vi "Total Analysis.vi"(6 "ROIIndex":i32, 7 "Algorithm":T1, 8 "error in":errorcluster, 9 "ROIList":string[][](array[string]), 10 "AlgParameter":string, 11 "Img in":T2) -> (0 "error out":errorcluster, 1 "DetectResult":variant, 2 "ResultOut":string[][](array[string]), 3 "Img out":T2)   [LabVIEW 2019]
uses:
  <vilib>/vision/Image Controls.llb/IMAQ Image.ctl
  Controls/V_Analysis_Type.ctl
  Controls/Analysis_Setting.ctl
  Ctrl/ROIDataType.ctl
  Controls/Parameter.ctl
  Controls/Color Pattern Match/Analysis Color Pattern Match Parameter.ctl
  Controls/Color Pattern Match/Analysis Color Pattern Match Result.ctl
  Controls/Parttern Match/Analysis_PatternMatch_Parameter.ctl
  Controls/ShapeDectect/Analysis_ShapeDectect_Parameter.ctl
  a7e08b04-c8a4-4d17-8d88-fa481432bc0a.vi
  bf7b5f5d-5c07-4b16-8f99-98f9c9cab738.vi
  dd62c550-2db8-45b5-a3de-447688dd18ca.vi
  c9a32d4f-7d2d-4bd1-920f-33aa71ed714f.vi
  4b400e5f-8bf9-44aa-89bd-445ffc1e469d.vi
  <vilib>/JDP Science/JSONtext/JSON text to Variant.vi
  <vilib>/vision/NI_Vision_Development_Module.lvlib
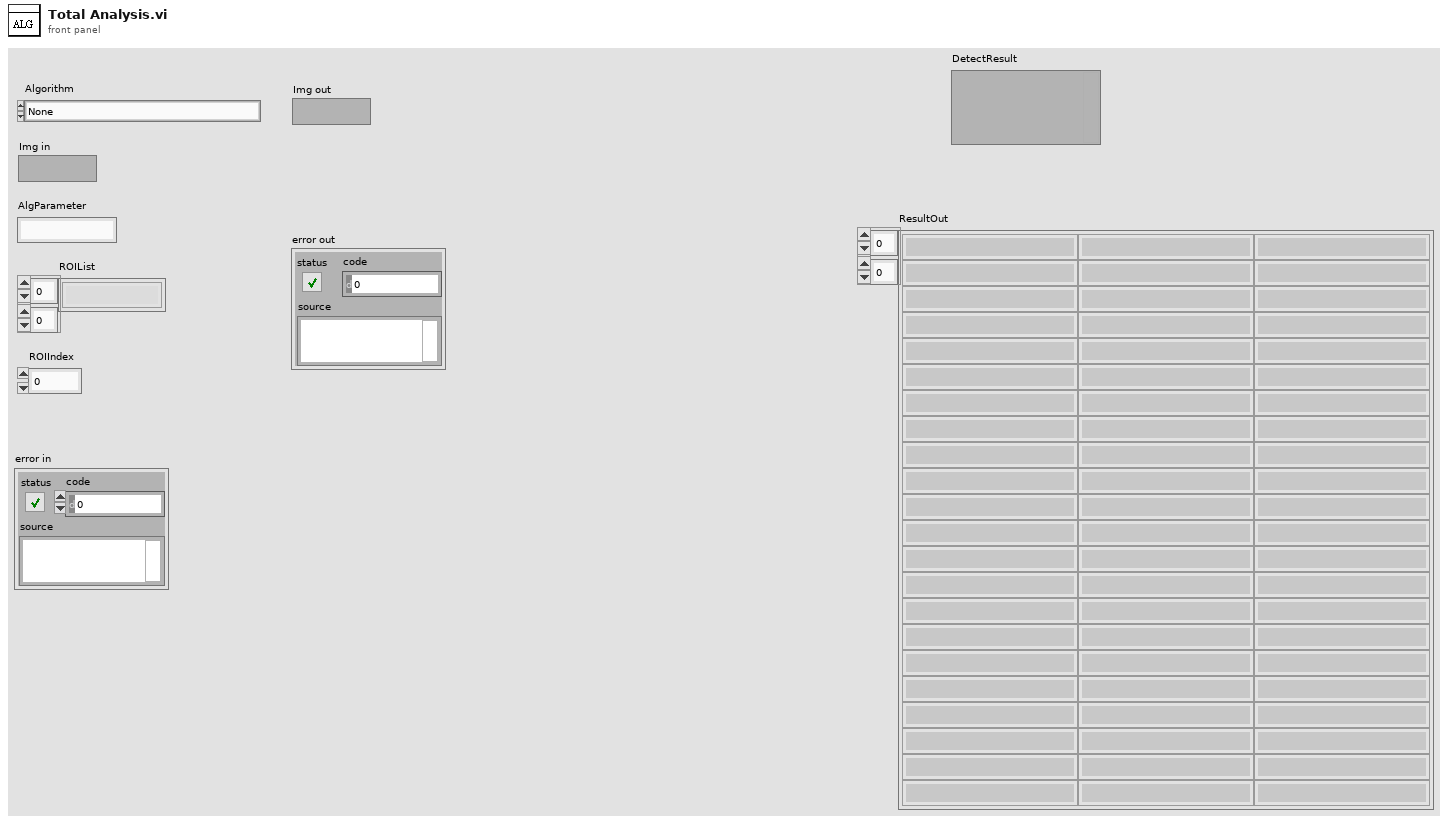
[diagram p1: front panel]
types:
  T1 = typedef "V_Analysis_Type.ctl" = enum16{"None", "C_Color Pattern Matching", "G_PatternMatching", "G_ShapeDectect", "G_GeometricMatch"}
  T2 = typedef "IMAQ Image.ctl" = refnum<image>
  T3 = typedef "Parameter.ctl" = enum16{"Initialize", "Write", "Read", "WriteAll", "Save", "Load"}
  T4 = typedef "ROIDataType.ctl" = cluster{"Global Rectangle":i32[], "Contours":cluster{"Contour Type":u32, "ROI Type":u32, "Points":i32[]}[]}
  T5 = typedef "Analysis Color Pattern Match Parameter.ctl" = cluster{"IgnoreBlack And White":enum16{"Disable", "IgnoreBlack", "IgnoreWhite", "IgnoreBlack And White"}, "Match Saturation Threshold":i32, "Minimum Match Score":i32, "Color Score Weight":i32, "Color Sensitivity":u32, "Search Strategy":u32, "Match Offset":cluster{"X":dbl, "Y":dbl}, "Number of Matches to Find":i32, "AngleRange+/-":dbl, "Sub-Pixel Accuracy":bool, "ROI Descriptor":T6, "TemplatePath":string, "Match Mode":enum16{"Shift Invariant", "Rotation Invariant"}}
  T6 = typedef "ROI Descriptor" = cluster{"Global Rectangle":i32[], "Contours":cluster{"ID":enum32{"External", "Internal"}, "Type":u32, "Coordinates":i32[]}[]}
  T7 = typedef "Analysis_ShapeDectect_Parameter.ctl" = cluster{"Enum_ShapeType":enum16{"Circles", "Ellipses", "Lines", "Rectangles"}, "MaxParticle":i32, "Descriptor":cluster{"Set 1":dbl, "Set 2":dbl, "Set 3":dbl, "Set 4":dbl}, "Match Options":cluster{"Rotation":bool, "Scale":bool, "Occlusion":bool, "Range Settings":cluster{"Match Constraints":u32, "Min":dbl, "Max":dbl}[]}, "Curve Parameters":cluster{"Extraction Mode":u32, "Edge Threshold":i32, "Edge Filter Size":u32, "Min Length":i32, "Row Search Step Size":i32, "Col Search Step Size":i32, "Max Endpoint Gap":i32, "Closed":bool, "Subpixel":bool}, " score":dbl}
  T8 = typedef "Analysis_Setting.ctl" = cluster{"PreProcess":T1, "Parameter":string}
  T9 = typedef "ParameterData.ctl" = cluster{"Rotate Angle":dbl, "Rotate?":bool, "Calibration File Path":string, "Cal?":bool}
  T10 = typedef "Image Type" = u32
  T11 = typedef "Analysis Color Pattern Match Result.ctl" = cluster{"Number of Matches":i32, "Matches out":cluster{"Position":cluster{"x":sgl, "y":sgl}, "Angle":sgl, "Scale":sgl, "Score":sgl, "Bounding Box":cluster{"x":sgl, "y":sgl}[]}[], "Calibrated Matches":cluster{"Position":cluster{"x":sgl, "y":sgl}, "Angle":sgl, "Scale":sgl, "Score":sgl, "Bounding Box":cluster{"x":sgl, "y":sgl}[]}[], "ROI Descriptor":T6}
  T12 = cluster{"Position":cluster{"x":sgl, "y":sgl}, "Angle":sgl, "Scale":sgl, "Score":sgl, "Bounding Box":cluster{"x":sgl, "y":sgl}[]}[]
  T13 = typedef "Analysis_PatternMatch_Parameter.ctl" = cluster{"Algorithm":i32, "Match Parameters":cluster{"Number of Matches Requested":i32, "Minimum Match Score":sgl, "Angle Ranges":cluster{"Start Angle":sgl, "End Angle":sgl}[]}, "ROI Descriptor":T6, "Advanced Options":cluster{"Item":u16, "Value":dbl}[], "Template path":string, "XOffset":i32, "YOffset":i32}
  T14 = typedef "Analysis_PatternMatch_Result.ctl" = cluster{"Position":cluster{"x":sgl, "y":sgl}, "Angle":sgl, "Scale":sgl, "Score":sgl, "Bounding Box":cluster{"x":sgl, "y":sgl}[]}
  T15 = cluster{"ResultOut":variant, "DectectItem":i32, "Data out":T4}
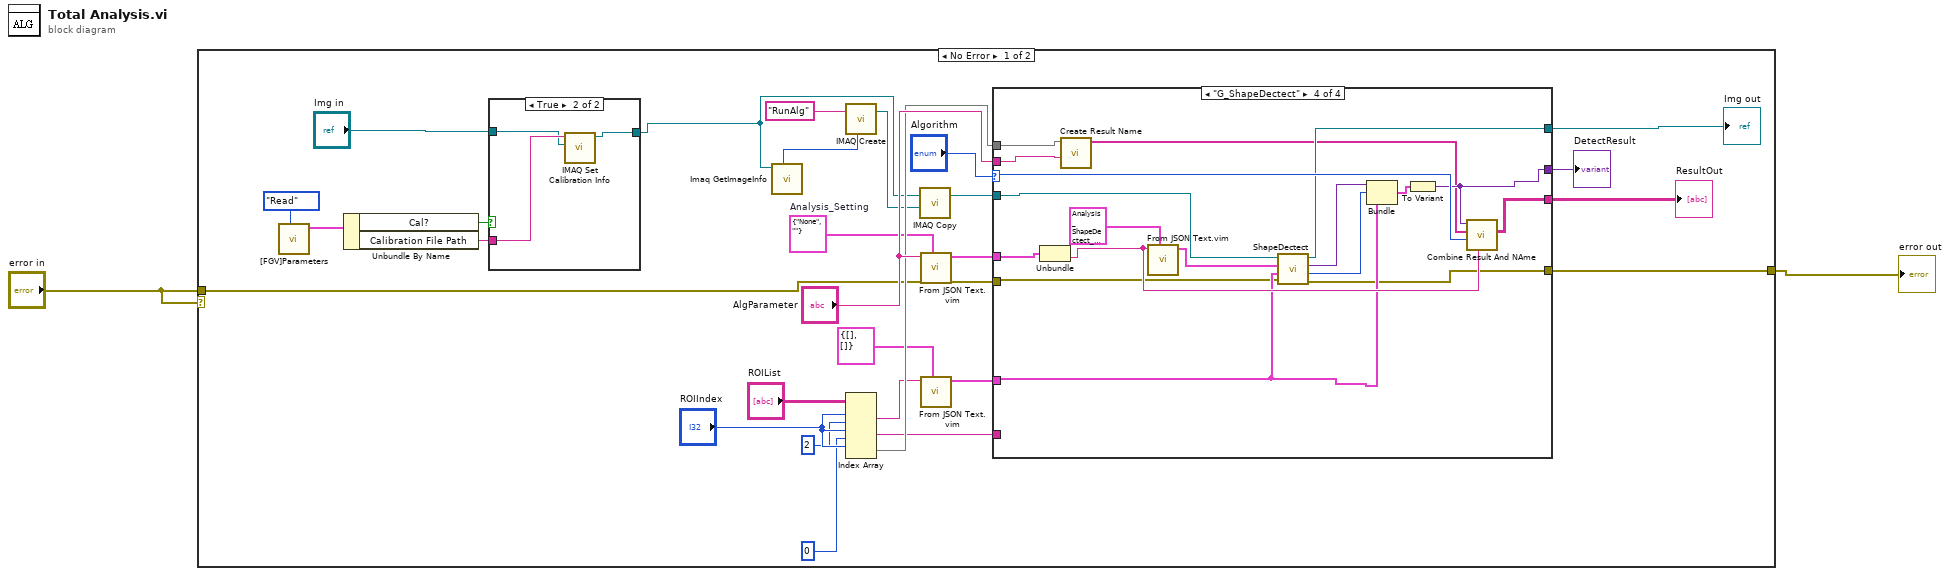
[diagram p0: block diagram]
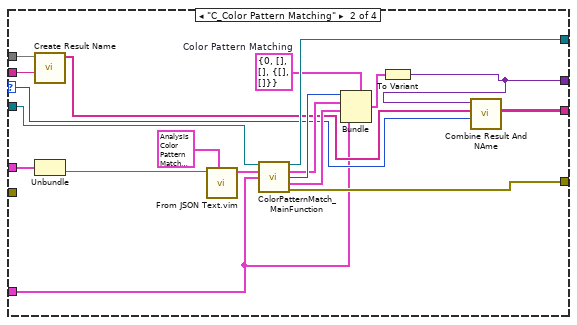
[diagram p4: hidden frame]
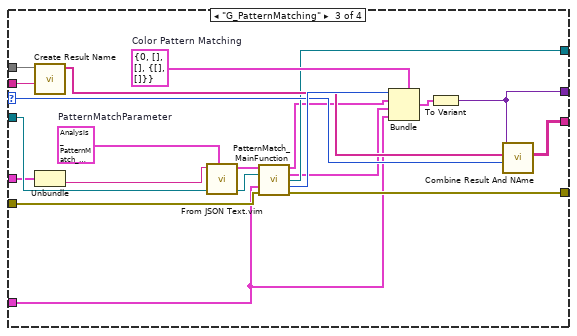
[diagram p5: hidden frame]
diagram:
  n1 = case shown="No Error" "error in" {
    tunnel: [w28 w92] -> w2
    tunnel: "error in" -> [w13 w92]
    frame No Error {
      w14 = T8 {"PreProcess"=enum."None", "Parameter"=""}  # Analysis_Setting
      n2 = call "[FGV]Parameters.vi"("Parameter"=Parameter."Read") -> ("ParameterData Out"=w7:T9)  [unwired: 9 in, 1 out]
      n3 = Unbundle By Name(w7) -> ("Cal?"=w6:bool, "Calibration File Path"=w5:string)
      n4 = case shown="True" w6 {
        tunnel: "Img in" -> [w31 w33]
        tunnel: w5 -> [_ w34]
        tunnel: [w31 w32] -> w3
        frame False {
        }
        frame True {
          n5 = call "IMAQ Set Calibration Info"("Image Dst"=w33, "Image Src"=w34) -> ("Calibrated Image"=w32:T2)  [unwired: 8 in, 1 out]
        }
      }
      n6 = call "Imaq GetImageInfo"("Image"=w3) -> ("Image Type"=w15:T10)  [unwired: 3 in, 7 out]
      n7 = call "IMAQ Create"("Image Name"="RunAlg", "Image Type"=w15) -> ("New Image"=w16:T2)  [unwired: 3 in, 1 out]
      n8 = Index Array(array="ROIList", index (row) #1="ROIIndex", index (col) #1=2 ("disabled index (col)"), index (row) #2="ROIIndex", index (col) #2=0 ("disabled index (col)"), index (row) #3="ROIIndex") -> (element #1=w21:string, element #2=w24:string, element #3=w27:string[])  [unwired: 1 in]
      n9 = call "IMAQ Copy"("Image Dst"=w16, "Image Src"=w3) -> ("Image Dst Out"=w18:T2)  [unwired: 4 in, 1 out]
      n10 = call "From JSON Text.vim"("Data Type and Default Value"=w14, "JSON"="AlgParameter") -> ("Data out"=w25:T8)  [unwired: 8 in, 1 out]
      n11 = call "From JSON Text.vim"("Data Type and Default Value"=T4 {"Global Rectangle"=[], "Contours"=[]} ("ROI DataType"), "JSON"=w21) -> ("Data out"=w22:T4)  [unwired: 8 in, 1 out]
      n12 = case shown="\"G_ShapeDectect\"" "Algorithm" {
        selector: "Algorithm" -> [_ w40 w65 w81]
        tunnel: w18 -> [_ w53 w73 w82]
        tunnel: w22 -> [_ w35 w56 w85]
        tunnel: [_ w52 w61 w80] -> w10
        tunnel: w24 -> [_ _ _ _]
        tunnel: w25 -> [_ w49 w71 w83]
        tunnel: w27 -> [_ w47 w70 w76]
        tunnel: [_ w42 w67 w77] -> w28
        tunnel: "AlgParameter" -> [_ w39 w64 w75]
        tunnel: [_ w38 w60 w78] -> w30
        tunnel: w13 -> [_ _ w59 w84]
        tunnel: [_ w36 w57 w79] -> w11
        frame "None", Default {
        }
        frame "C_Color Pattern Matching" {
          w46 = T11 {"Number of Matches"=0, "Matches out"=[], "Calibrated Matches"=[], "ROI Descriptor"={"Global Rectangle"=[], "Contours"=[]}}  # Color Pattern Matching
          n13 = call "Create Result Name.vi"("AlgSet"=w39, "ROIList"=w47) -> ("AlgResultName"=w41:string[])  [unwired: 9 in]
          n14 = Unbundle(w49) -> ("Parameter"=w51:string)  [unwired: 1 out]
          n15 = call "From JSON Text.vim"("Data Type and Default Value"=T5 {"IgnoreBlack And White"=enum."IgnoreBlack And White", "Match Saturation Threshold"=80, "Minimum Match Score"=750, "Color Score Weight"=750, "Color Sensitivity"=1, "Search Strategy"=0, "Match Offset"={"X"=0.0, "Y"=0.0}, "Number of Matches to Find"=0, "AngleRange+/-"=0.0, "Sub-Pixel Accuracy"=FALSE, "ROI Descriptor"={"Global Rectangle"=[], "Contours"=[]}, "TemplatePath"="", "Match Mode"=enum."Rotation Invariant"} ("Color Pattern Match"), "JSON"=w51) -> ("Data out"=w48:T5)  [unwired: 8 in, 1 out]
          n16 = call "ColorPatternMatch_MainFunction.vi"("Image in"=w53, "Color Pattern Match"=w48, "ROI Descriptor"=w35) -> ("Image Out"=w52:T2, "Matches out"=w44:T12, "Number of Matches"=w45:i32, "Calibrated Matches"=w43:T12, "error out"=w42:errorcluster)  [unwired: 8 in]
          n17 = Bundle(cluster=w46, "Number of Matches"=w45, "Matches out"=w44, "Calibrated Matches"=w43, "ROI Descriptor"=w35) -> (w37:T11)
          n18 = To Variant(anything=w37) -> (Variant=w36:variant)
          n19 = call "Combine Result And NAme.vi"("Analysis"=w40, "AlgResultName"=w41, "DataIn"=w36) -> ("ResultOut"=w38:string[][])  [unwired: 8 in]
        }
        frame "G_PatternMatching" {
          w63 = T13 {"Algorithm"=2, "Match Parameters"={"Number of Matches Requested"=1, "Minimum Match Score"=750.0, "Angle Ranges"=[]}, "ROI Descriptor"={"Global Rectangle"=[], "Contours"=[]}, "Advanced Options"=[{"Item"=1, "Value"=1.0}, {"Item"=103, "Value"=1.0}], "Template path"="", "XOffset"=0, "YOffset"=0}  # PatternMatchParameter
          w69 = T11 {"Number of Matches"=0, "Matches out"=[], "Calibrated Matches"=[], "ROI Descriptor"={"Global Rectangle"=[], "Contours"=[]}}  # Color Pattern Matching
          n20 = call "Create Result Name.vi"("AlgSet"=w64, "ROIList"=w70) -> ("AlgResultName"=w66:string[])  [unwired: 9 in]
          n21 = Unbundle(w71) -> ("Parameter"=w72:string)  [unwired: 1 out]
          n22 = call "From JSON Text.vim"("Data Type and Default Value"=w63, "JSON"=w72) -> ("Data out"=w62:T13)  [unwired: 8 in, 1 out]
          n23 = call "PatternMatch_MainFunction.vi"("PatternMatchParameter"=w62, "Vision_Image In"=w73, "ROI Descriptor"=w56, "error in"=w59) -> ("Matches"=w55:T14[], "Matches (real-world)"=w54:T12, "Image (duplicate)"=w61:T2, "Number of Matches"=w68:i32, "error out"=w67:errorcluster)  [unwired: 7 in]
          n24 = Bundle(cluster=w69, "Number of Matches"=w68, "Matches out"=w55, "Calibrated Matches"=w54, "ROI Descriptor"=w56) -> (w58:T11)
          n25 = To Variant(anything=w58) -> (Variant=w57:variant)
          n26 = call "Combine Result And NAme.vi"("Analysis"=w65, "AlgResultName"=w66, "DataIn"=w57) -> ("ResultOut"=w60:string[][])  [unwired: 8 in]
        }
        frame "G_ShapeDectect" {
          n27 = Unbundle(w83) -> ("Parameter"=w86:string)  [unwired: 1 out]
          n28 = call "Create Result Name.vi"("AlgSet"=w75, "ROIList"=w76) -> ("AlgResultName"=w74:string[])  [unwired: 9 in]
          n29 = call "From JSON Text.vim"("Data Type and Default Value"=T7 {"Enum_ShapeType"=enum."Circles", "MaxParticle"=1, "Descriptor"={"Set 1"=100.0, "Set 2"=10.0, "Set 3"=200.0, "Set 4"=10.0}, "Match Options"={"Rotation"=TRUE, "Scale"=FALSE, "Occlusion"=FALSE, "Range Settings"=[{"Match Constraints"=0, "Min"=0.0, "Max"=360.0}]}, "Curve Parameters"={"Extraction Mode"=0, "Edge Threshold"=75, "Edge Filter Size"=1, "Min Length"=25, "Row Search Step Size"=15, "Col Search Step Size"=15, "Max Endpoint Gap"=10, "Closed"=FALSE, "Subpixel"=FALSE}, " score"=500.0} ("SetParameter"), "JSON"=w86) -> ("Data out"=w88:T7)  [unwired: 8 in, 1 out]
          n30 = call "ShapeDectect.vi"("error in (no error)"=w84, "ROI Descriptor"=w85, "SetParameter"=w88, "Image In"=w82) -> ("error out"=w77:errorcluster, "DectectItem"=w87:i32, "ResultOut"=w91:variant, "Image Out"=w80:T2)  [unwired: 4 in]
          n31 = Bundle("ResultOut"=w91, "DectectItem"=w87, "Data out"=w85) -> (w90:T15)  [unwired: 1 in]
          n32 = To Variant(anything=w90) -> (Variant=w79:variant)
          n33 = call "Combine Result And NAme.vi"("SetParameter"=w86, "Analysis"=w81, "AlgResultName"=w74, "DataIn"=w79) -> ("ResultOut"=w78:string[][])  [unwired: 7 in]
        }
      }
      "ResultOut" <- w30
      "Img out" <- w10
      "DetectResult" <- w11
    }
    frame Error {
    }
  }
  "error out" <- w2
